vi "Parse Sorted Object Dictionary.vi"(8 "error in":errorcluster, 11 "reference in":refnum<class "Electronic Datasheet.lvclass">) -> (0 "error out":errorcluster, 3 "reference out":refnum<class "Electronic Datasheet.lvclass">)   [LabVIEW 2024, in "Electronic Datasheet.lvlib" / "Electronic Datasheet.lvclass"]
uses:
  Electronic Datasheet.lvclass
  Core/Sorted Object Dictionary/Sorted Object Dictionary.lvclass
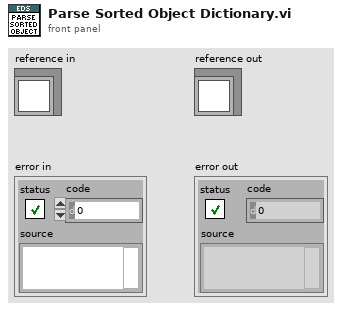
[diagram p1: front panel]
types:
  T1 = typedef "Electronic Datasheet.lvlib/Electronic Datasheet.lvclass/ObjectAttributes.ctl" = cluster{"EDS File Path":path, "Object Dict":refnum<class "Dictionary.lvclass">, "Sorted Object Dict":refnum<class "Sorted Object Dictionary.lvclass">, "Device Info":refnum<class "Device Info.lvclass">, "File Info":refnum<class "File Info.lvclass">}
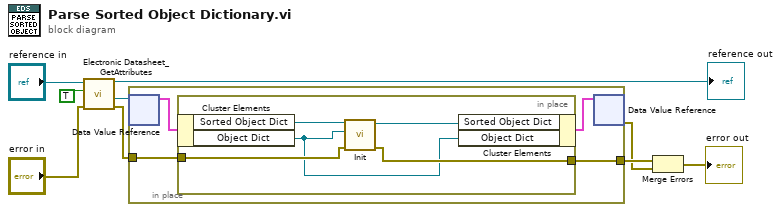
[diagram p0: block diagram]
diagram:
  n1 = call "Electronic Datasheet_GetAttributes.vi"("Error In"="error in", "OnlyGetDvrReference(False)"=TRUE, "reference in"="reference in") -> ("Error Out"=w5:errorcluster, "DataRef"=w6:refnum<data-value>, "reference out"=→"reference out":refnum<class "Electronic Datasheet.lvclass">)  [unwired: 5 in, 1 out]
  n2 = in-place {
    in-place-border: w5 -> [w12]
    in-place-border: [w11] -> w4
    n3 = in-place-dvr #1(w6) -> (w13:T1)  [unwired: 1 out]
    n4 = in-place {
      in-place-border: w12 -> [w17]
      in-place-border: [w16] -> w11
      n5 = in-place-cluster #2(w13) -> ("Sorted Object Dict"=w18:refnum<class "Sorted Object Dictionary.lvclass">, "Object Dict"=w14:refnum<class "Dictionary.lvclass">)
      n6 = call "Init.vi"("error in"=w17, "Dictionary"=w14, "Sorted Object Dictionary in"=w18) -> ("error out"=w16:errorcluster, "Sorted Object Dictionary out"=w15:refnum<class "Sorted Object Dictionary.lvclass">)  [unwired: 7 in]
      n7 = in-place-cluster #2("Sorted Object Dict"=w15, "Object Dict"=w14) -> (w10:T1)
    }
    n8 = in-place-dvr #1(w10) -> (w3:errorcluster)  [unwired: 1 out]
  }
  n9 = Merge Errors(w4, w3) -> (→"error out":errorcluster)
